vi "Curtin_MicErrorCheck.vi"(8 "error in (no error)":errorcluster) -> ()   [LabVIEW 2022 SP3]
uses:
  <vilib>/Utility/error.llb/DialogType.ctl
panel:
  out "code":i32
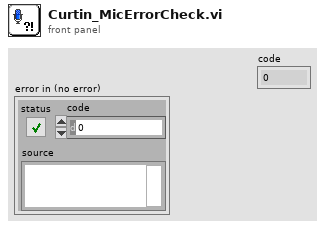
[diagram p1: front panel]
types:
  T1 = typedef "DialogType.ctl" = u16
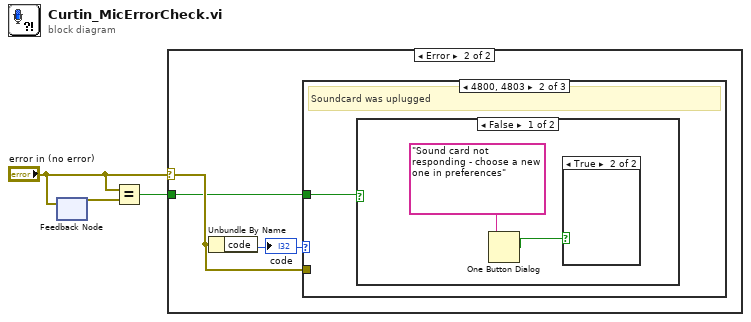
[diagram p0: block diagram]
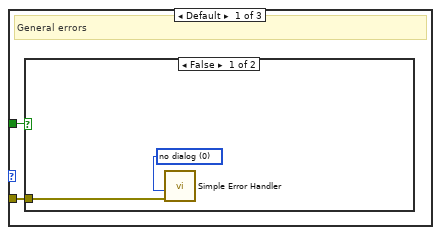
[diagram p3: hidden frame]
diagram:
  n1 = feedback-in #1("error in (no error)") -> ()
  n2 = feedback #1() -> (w3:errorcluster)  [unwired: 1 in]
  n3 = Equal?(x="error in (no error)", y=w3) -> (x = y?=w1:bool)
  n4 = case shown="Error" "error in (no error)" {
    selector: "error in (no error)" -> [_ w5]
    tunnel: w1 -> [_ w4]
    frame No Error {
    }
    frame Error {
      n5 = Unbundle By Name(w5) -> ("code"=w6:i32)
      "code" <- w6
      n6 = case shown="4800, 4803" w6 {
        tunnel: w5 -> [w8 _ _]
        tunnel: w4 -> [w7 w11 _]
        frame Default {
          # "General errors"
          n7 = case shown="False" w7 {
            tunnel: w8 -> [w9 _]
            frame False {
              w10 = T1 0 items=["no dialog", "OK message", "continue or stop message", "OK message + warnings", "continue/stop + warnings"] ("type of dialog (OK msg:1)")
              n8 = call <vilib>:"Simple Error Handler.vi"("type of dialog (OK msg:1)"=w10, "error in (no error)"=w9) -> ()  [unwired: 3 in, 5 out]
            }
            frame True {
            }
          }
        }
        frame 4800, 4803 {
          # "Soundcard was uplugged"
          n9 = case shown="False" w11 {
            frame False {
              n10 = One Button Dialog(message="Sound card not responding - choose a new one in preferences") -> (true=w12:bool)  [unwired: 1 in]
              n11 = case shown="True" w12 {
                frame False {
                }
                frame True {
                }
              }
            }
            frame True {
            }
          }
        }
        frame 4822 {
          # "Timed out grabbing data"
        }
      }
    }
  }
